vi "Gyro Setup.vi"(8 "error in":errorcluster, 11 "Yaw in":dbl) -> (3 "Yaw Out":dbl)   [LabVIEW 2016]
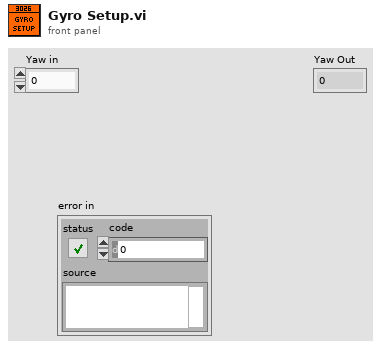
[diagram p1: front panel]
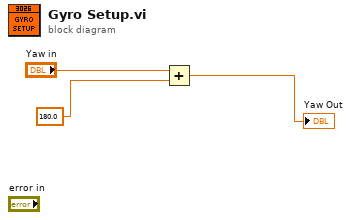
[diagram p0: block diagram]
diagram:
  n1 = Add(x="Yaw in", y=180.0) -> (x+y=→"Yaw Out":dbl)
